vi "CompTrigStopProps.vi"(0 "task in":refnum<k24>, 5 "error in (no error)":errorcluster) -> (8 "TriggerChannelStr":string, 9 "AnalogSWTriggerSense":i32, 10 "TriggerChannel":i32, 11 "CounterChannelTriggerSense":i32, 12 "Variance":dbl, 13 "DigitalPatternTriggerSense":i32, 14 "task out":refnum<k24>, 15 "Level":dbl, 16 "Type":i32, 19 "error IO":errorcluster)   [LabVIEW 2010]
uses:
  C:/Program Files/National Instruments/LabVIEW 2010/vi.lib/ULx/ULx_LV.dll
  Program Files/National Instruments/LabVIEW 2010/vi.lib/ULx/ULx_LV.dll
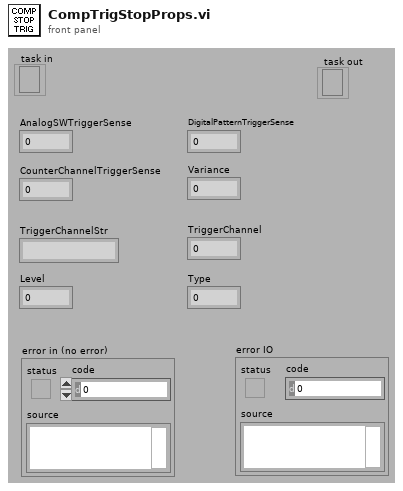
[diagram p1: front panel]
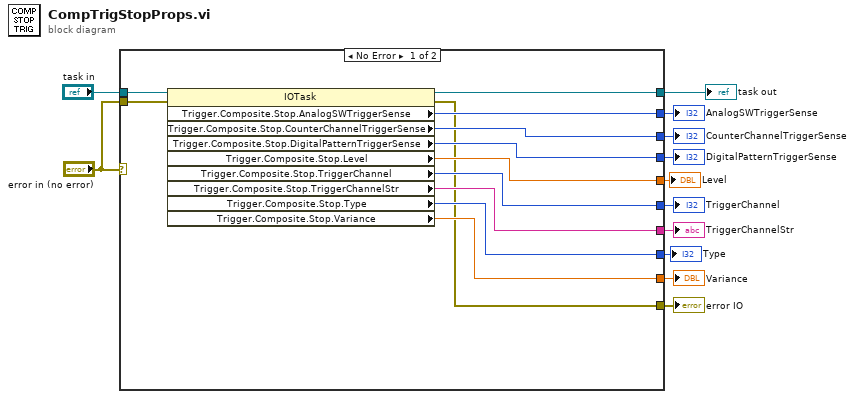
[diagram p0: block diagram]
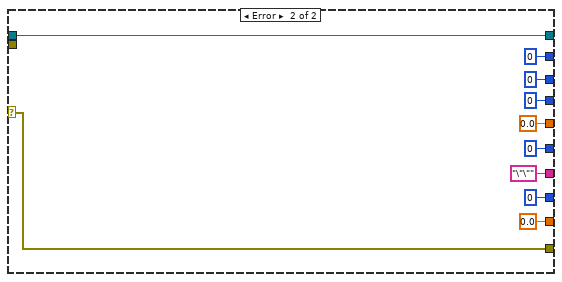
[diagram p2: hidden frame]
diagram:
  n1 = case shown="No Error" "error in (no error)" {
    selector: "error in (no error)" -> [_ w33]
    tunnel: "task in" -> [w24 w34]
    tunnel: "error in (no error)" -> [w23 _]
    tunnel: [w22 w34] -> w10
    tunnel: [w21 0 ("Trigger.Composite.Stop.AnalogSWTriggerSense")] -> w9
    tunnel: [w20 0 ("Trigger.Composite.Stop.CounterChannelTriggerSense")] -> w8
    tunnel: [w19 0 ("Trigger.Composite.Stop.DigitalPatternTriggerSense")] -> w7
    tunnel: [w18 0.0 ("Trigger.Composite.Stop.Level")] -> w6
    tunnel: [w17 0 ("Trigger.Composite.Stop.TriggerChannel")] -> w5
    tunnel: [w16 "\"\"" ("Trigger.Composite.Stop.TriggerChannelStr")] -> w4
    tunnel: [w15 0 ("Trigger.Composite.Stop.Type")] -> w3
    tunnel: [w14 0.0 ("Trigger.Composite.Stop.Variance")] -> w2
    tunnel: [w13 w33] -> w1
    frame No Error {
      n2 = property class="IOTask"(reference=w24, error in=w23) -> (reference out=w22:refnum<k24>, error out=w13:errorcluster, "Trigger.Composite.Stop.AnalogSWTriggerSense"=w21:i32, "Trigger.Composite.Stop.CounterChannelTriggerSense"=w20:i32, "Trigger.Composite.Stop.DigitalPatternTriggerSense"=w19:i32, "Trigger.Composite.Stop.Level"=w18:dbl, "Trigger.Composite.Stop.TriggerChannel"=w17:i32, "Trigger.Composite.Stop.TriggerChannelStr"=w16:string, "Trigger.Composite.Stop.Type"=w15:i32, "Trigger.Composite.Stop.Variance"=w14:dbl)
    }
    frame Error {
    }
  }
  "task out" <- w10
  "AnalogSWTriggerSense" <- w9
  "CounterChannelTriggerSense" <- w8
  "DigitalPatternTriggerSense" <- w7
  "Level" <- w6
  "TriggerChannel" <- w5
  "TriggerChannelStr" <- w4
  "Type" <- w3
  "Variance" <- w2
  "error IO" <- w1
